vi "Write Return Address.vi"(10 "Return Address":refnum<class "Message Enqueuer.lvclass">, 11 "PreAddressedMsg in":refnum<class "PreAddressedMsg.lvclass">) -> (3 "PreAddressedMsg out":refnum<class "PreAddressedMsg.lvclass">)   [LabVIEW 2015, in "AbstractMessages.lvlib" / "PreAddressedMsg.lvclass"]
uses:
  PreAddressedMsg.lvclass
  <vilib>/ActorFramework/Message Enqueuer/Message Enqueuer.lvclass
  PreAddressedMsg.lvclass/PreAddressedMsg.ctl
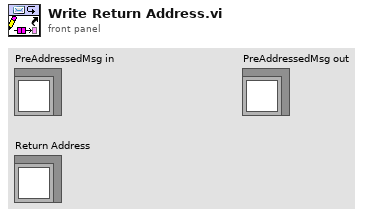
[diagram p1: front panel]
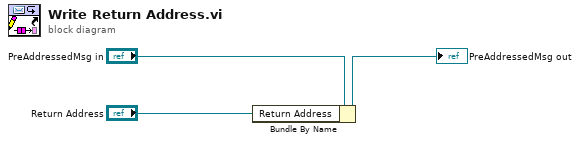
[diagram p0: block diagram]
diagram:
  n1 = Bundle By Name(cluster="PreAddressedMsg in", "Return Address"="Return Address") -> (→"PreAddressedMsg out":refnum<class "PreAddressedMsg.lvclass">)
